vi "KGV.vi"(11 "Array":u64[](array[numeric])) -> (3 "KGV":u64)   [LabVIEW 2021]
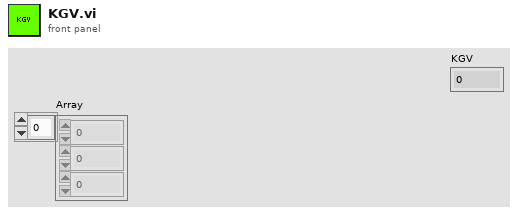
[diagram p1: front panel]
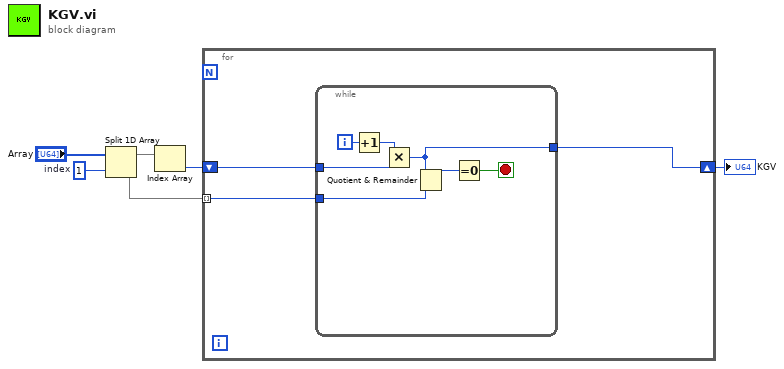
[diagram p0: block diagram]
diagram:
  w5 = 1  # index
  n1 = Split 1D Array(array="Array", index=w5) -> (first subarray=w4:u64[], second subarray=w2:u64[])
  n2 = Index Array(array=w4) -> (element=w3:u64)  [unwired: 1 in]
  n3 = for {
    tunnel: w2 -> [w8] mode=indexing
    shift-right: [w7] -> w1
    shift-left: w3 -> [w9]
    n4 = while {
      tunnel: w9 -> [w16]
      tunnel: w8 -> [w13]
      tunnel: [w10] -> w7
      i -> [w15]
      stop <- w11 stop-if-true
      n5 = Increment(x=w15) -> (x+1=w14:i32)
      n6 = Multiply(x=w14, y=w16) -> (x*y=w10:u64)
      n7 = Quotient & Remainder(x=w10, y=w13) -> (x-y*floor(x/y)=w12:u64)  [unwired: 1 out]
      n8 = Equal To 0?(x=w12) -> (x = 0?=w11:bool)
    }
  }
  "KGV" <- w1
